vi "Queue auf Log File schreiben vorbereiten.vi"(10 "Queue":refnum<queue>) -> (2 "Queue":refnum<queue>)   [LabVIEW 2020, in "LogKonfig.lvlib"]
uses:
  LogKonfig.lvlib
  FT-IR/TOOLweb Interface Library/TOOLweb Signalverlaeufe.ctl
  Aktionen Trigger.ctl
  FT-IR/TOOLweb Interface Library/Typdefinitionen.lvlib
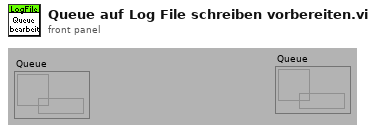
[diagram p1: front panel]
types:
  T1 = typedef "LogKonfig.lvlib/Aktionen Trigger.ctl" = enum16{"lesen", "ALLE schreiben", "Trigger prüfen", "Trigger rücksetzen"}
  T2 = typedef "LogKonfig.lvlib/Element Triggerereignisse.ctl" = cluster{"Trigger verwenden":T3, "Messwert":u16, "kl./gr.":u16, "Wert":sgl, "Puffergröße":sgl}
  T3 = typedef "LogKonfig.lvlib/Auswahlfeld aktiviert-deaktiviert.ctl" = u16
  T4 = typedef "FT-IR.lvlib/TOOLweb Interface.lvlib/Typdefinitionen.lvlib/TOOLweb Signalverlaeufe.ctl" = waveform(dbl)[]
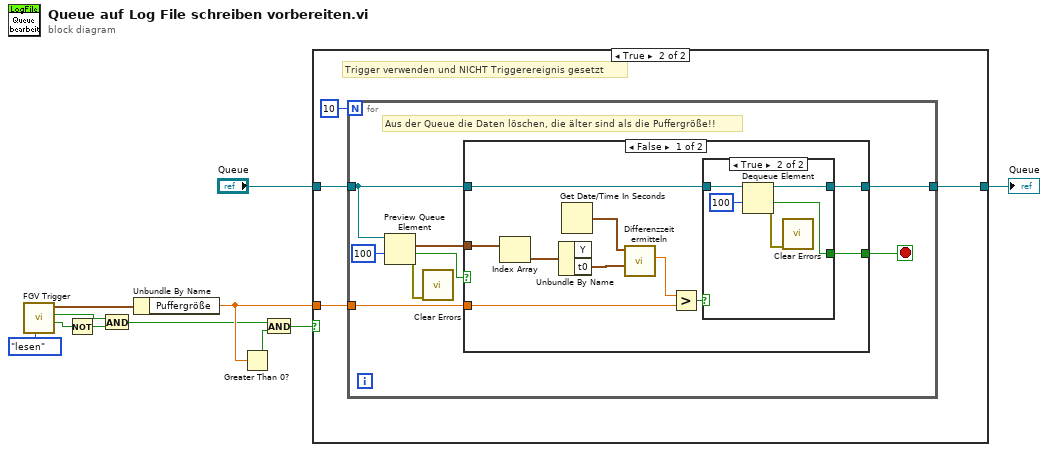
[diagram p0: block diagram]
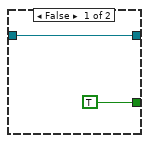
[diagram p3: hidden frame]
diagram:
  n1 = call "FGV Trigger.vi"("Aktion"=Aktionen_Trigger."lesen") -> ("Trigger gesetzt?"=w6:bool, "Trigger verwenden"=w7:bool, "Triggerereignis neu"=w5:T2)  [unwired: 7 in, 1 out]
  n2 = Not(x=w6) -> (.not. x?=w8:bool)
  n3 = And(x=w7, y=w8) -> (x .and. y?=w2:bool)
  n4 = Unbundle By Name(w5) -> ("Puffergröße"=w4:sgl)
  n5 = Greater Than 0?(x=w4) -> (x > 0?=w3:bool)
  n6 = And(x=w2, y=w3) -> (x .and. y?=w1:bool)
  n7 = case shown="True" w1 {
    tunnel: "Queue" -> [w12 w16]
    tunnel: [w12 w15] -> w9
    tunnel: w4 -> [_ w13]
    frame False {
      # "Trigger nicht verwenden\nODER\nTrigger verwenden aber Trigerereignis aktiv"
    }
    frame True {
      # "Trigger verwenden und NICHT Triggerereignis gesetzt"
      n8 = for {
        N: 10 -> [_]
        tunnel: w16 -> [w21]
        tunnel: [w20] -> w15
        tunnel: w13 -> [w18]
        stop <- w19 stop-if-true
        # "Aus der Queue die Daten löschen, die älter sind als die Puffergröße!!"
        n9 = Preview Queue Element(queue=w21, timeout in ms (-1)=100 ("Timeout in ms(-1)")) -> (element=w22:T4, timed out?=w23:bool, error out=w17:errorcluster)  [unwired: 1 in, 1 out]
        n10 = call <vilib>:"Clear Errors.vi"("error in (no error)"=w17) -> ()  [unwired: 5 in, 2 out]
        n11 = case shown="False" w23 {
          selector: w23 -> [_ w42]
          tunnel: w22 -> [w34 _]
          tunnel: w21 -> [w28 w43]
          tunnel: [w27 w43] -> w20
          tunnel: [w26 w42] -> w19
          tunnel: w18 -> [w25 _]
          frame False {
            n12 = Index Array(array=w34) -> (element=w33:waveform(dbl))  [unwired: 1 in]
            n13 = Unbundle By Name(w33) -> ("t0"=w31:timestamp)  [unwired: 1 out]
            n14 = Get Date/Time In Seconds() -> (seconds since 1Jan1904=w32:timestamp)
            n15 = call "Differenzzeit ermitteln.vi"("Zeitstempel 2"=w31, "Zeitstempel 1"=w32) -> ("Differenzzeit in sec"=w30:sgl)  [unwired: 8 in, 1 out]
            n16 = Greater?(x=w30, y=w25) -> (0:w29:bool)
            n17 = case shown="True" w29 {
              tunnel: w28 -> [w35 w41]
              tunnel: [w35 w40] -> w27
              tunnel: [TRUE ("timed out?") w38] -> w26
              frame False {
              }
              frame True {
                n18 = Dequeue Element(queue=w41, timeout in ms (-1)=100 ("Timeout in ms(-1)")) -> (queue out=w40:refnum<queue>, timed out?=w38:bool, error out=w37:errorcluster)  [unwired: 1 in, 1 out]
                n19 = call <vilib>:"Clear Errors.vi"("error in (no error)"=w37) -> ()  [unwired: 5 in, 2 out]
              }
            }
          }
          frame True {
          }
        }
      }
    }
  }
  "Queue" <- w9
